vi "Disabled.vi"(7 "Robot Mode":T2, 10 "Match Info":T1={"Autonomous Elapsed Seconds"=0.0, "TeleOp Elapsed Seconds"=0.0, "Disabled Elapsed Seconds"=0.0, "Visited Autonomous"=FALSE, "Visited TeleOp"=FALSE, "Visited Disabled"=FALSE, "Autonomous Settings"={"Autonomous Style"=enum."Independent", "VI Refnum"=refnum}}, 11 "Call Context":T3) -> ()   [LabVIEW 2011]
doc: "This VI is called each time a disabled packet is received from the DS. It is often used to prepare for the next robot mode, to calibrate sensors, etc."
uses:
  <vilib>/Rock Robotics/WPI/DriverStation/WPI_DriverStationDerivedRobotMode.ctl
  <vilib>/Rock Robotics/WPI/DriverStation/WPI_DriverStationRobotMode.ctl
  <vilib>/Rock Robotics/WPI/DriverStation/WPI_DriverStationMatch Info.ctl
  <vilib>/Rock Robotics/WPI/DriverStation/DriverStationLCD/WPI_DriverStationLCDLCDLine.ctl
  <vilib>/Rock Robotics/WPI/CAN/Jaguar/SubVIs/WPI_CANJaguar_ControlMode.ctl
  <vilib>/Rock Robotics/WPI/MotorControl/WPI_MotorControlDeviceRef.ctl
  <vilib>/Rock Robotics/SystemInterfaces/Typedef/FPGA_TypedefDigitalModule.ctl
  <vilib>/Rock Robotics/SystemInterfaces/DIO/FPGA_DIOPWMChannel.ctl
  <vilib>/Rock Robotics/WPI/PWM/WPI_PWMDeadband.ctl
  <vilib>/Rock Robotics/WPI/PWM/WPI_PWMTransform_ConPane.ctl
  <vilib>/Utility/file.llb/Read From Spreadsheet File (string).vi
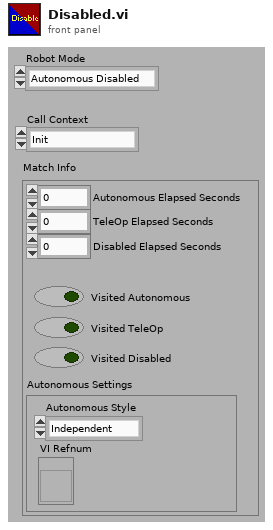
[diagram p1: front panel]
types:
  T1 = typedef "WPI_DriverStationMatch Info.ctl" = cluster{"Autonomous Elapsed Seconds":dbl, "TeleOp Elapsed Seconds":dbl, "Disabled Elapsed Seconds":dbl, "Visited Autonomous":bool, "Visited TeleOp":bool, "Visited Disabled":bool, "Autonomous Settings":cluster{"Autonomous Style":enum16{"Iterative", "Independent"}, "VI Refnum":refnum<vi>}}
  T2 = typedef "WPI_DriverStationRobotMode.ctl" = enum16{"Autonomous Disabled", "Autonomous Enabled", "Teleop Disabled", "Teleop Enabled", "Timeout", "Finish"}
  T3 = typedef "WPI_DriverStationDerivedRobotMode.ctl" = enum16{"Init", "Execute", "Stop"}
  T4 = typedef "WPI_MotorControlDeviceRef.ctl" = cluster{"DeviceStatus":errorcluster, "Type":enum16{"PWM", "CAN"}, "PWM":cluster{"Digital Module":T5, "PWM Channel":T6, "DeadBand":T7}, "CAN":cluster{"Device Number":u8, "Control Mode":T8, "Semaphore":T9, "Max Vout":dbl}, "Invert":bool, "TransformRef":T10, "InvTransformRef":T10}
  T5 = typedef "FPGA_TypedefDigitalModule.ctl" = enum16{"Digital Module 1", "Digital Module 2"}
  T6 = typedef "FPGA_DIOPWMChannel.ctl" = enum8{"PWM 1", "PWM 2", "PWM 3", "PWM 4", "PWM 5", "PWM 6", "PWM 7", "PWM 8", "PWM 9", "PWM 10", "Invalid"}
  T7 = typedef "WPI_PWMDeadband.ctl" = cluster{"Name":string, "maxPositivePwm":i32, "minPositivePwm":i32, "centerPwm":i32, "maxNegativePwm":i32, "minNegativePwm":i32, "angularRange":u16}
  T8 = typedef "WPI_CANJaguar_ControlMode.ctl" = enum8{"Percent VBus", "Current", "Speed", "Position", "Voltage"}
  T9 = typedef "Semaphore RefNum" = refnum<k1>
  T10 = typedef "WPI_PWMTransform_ConPane.ctl" = refnum<vi>
  T11 = typedef "WPI_DriverStationLCDLCDLine.ctl" = enum16{"Main - Line 1", "User - Line 2", "User - Line 3", "User - Line 4", "User - Line 5", "User - Line 6"}
  T12 = typedef "WPI_JoystickDevRef.ctl" = cluster{"Device":T13}
  T13 = typedef "WPI_JoystickDeviceEnum.ctl" = enum16{"USB 1", "USB 2", "USB 3", "USB 4", "Kinect 1", "Kinect 2"}
  T14 = typedef "WPI_JoystickButtonState.ctl" = cluster{"Button 1":bool, "Button 2":bool, "Button 3":bool, "Button 4":bool, "Button 5":bool, "Button 6":bool, "Button 7":bool, "Button 8":bool, "Button 9":bool, "Button 10":bool, "Button 11":bool, "Button 12":bool}
  T15 = cluster{"axis 1 (x)":dbl, "axis 2 (y)":dbl, "axis 3 (throttle)":dbl, "axis 4":dbl, "axis 5":dbl, "axis 6":dbl}
  T16 = typedef "IMAQ Image.ctl" = refnum<image>
  T17 = enum32{"Gray", "Binary", "Gradient", "Rainbow", "Temperature"}
  T18 = typedef "WPI_CameraDevRef.ctl" = cluster{"Camera Address":string, "CameraStatus":errorcluster, "Acquire Image Notifier":refnum<notifier>}
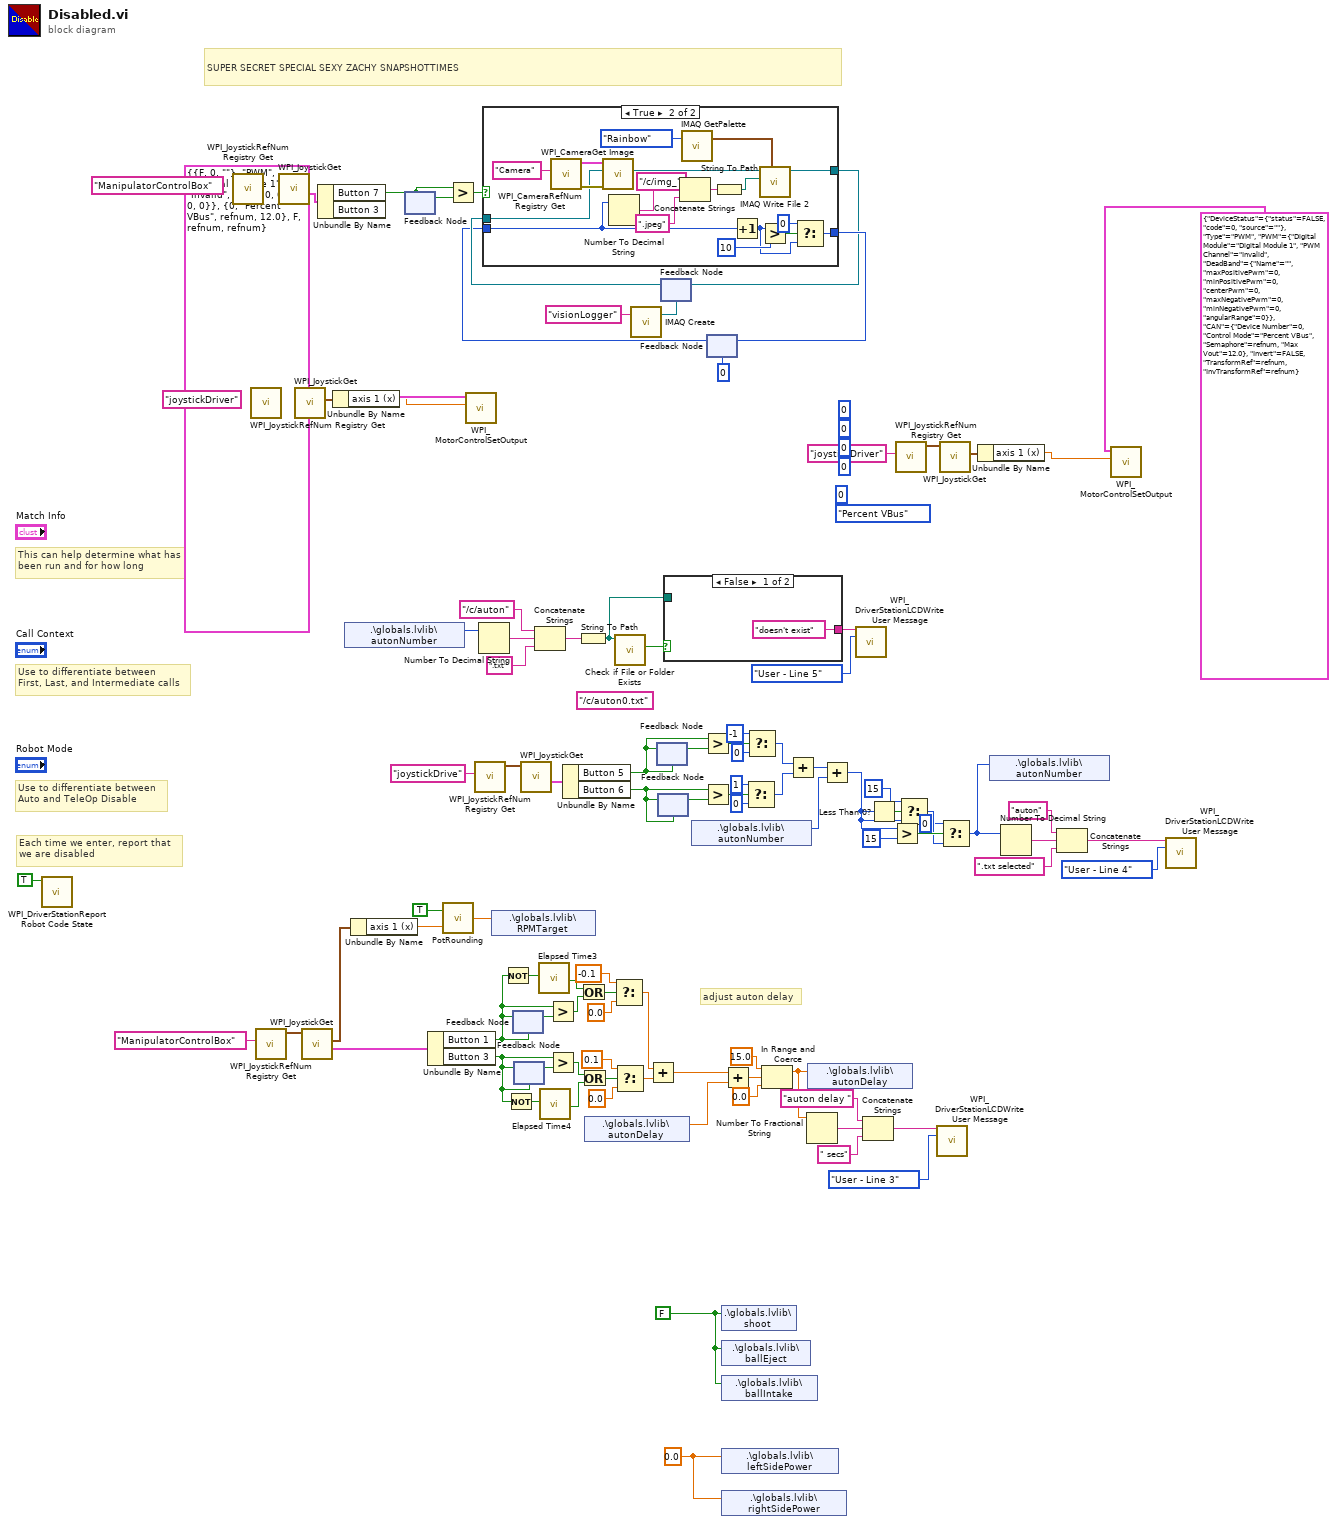
[diagram p0: block diagram]
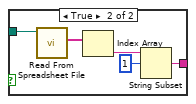
[diagram p3: hidden frame]
diagram:
  (unwired) 0 ("centerPwm")
  (unwired) 0 ("maxNegativePwm")
  (unwired) 0 ("minNegativePwm")
  (unwired) u16 0 ("angularRange")
  (unwired) u8 0 ("Device Number")
  (unwired) WPI_CANJaguar_ControlMode."Percent VBus" ("Control Mode")
  w29 = 0.0 ("leftSidePower")
  (unwired) "/c/auton0.txt" ("f")
  w100 = FALSE ("shoot")
  # "SUPER SECRET SPECIAL SEXY ZACHY SNAPSHOTTIMES"
  # "adjust auton delay"
  # "Each time we enter, report that\nwe are disabled"
  # "Use to differentiate between\nFirst, Last, and Intermediate calls"
  # "This can help determine what has\nbeen run and for how long"
  # "Use to differentiate between\nAuto and TeleOp Disable"
  n1 = call <vilib>:"WPI_DriverStationReport Robot Code State.vi"("Disabled"=TRUE ("Autonomous")) -> ()  [unwired: 10 in, 1 out]
  n2 = call <vilib>:"WPI_JoystickRefNum Registry Get.vi"("refnum name"="ManipulatorControlBox") -> ("JoystickDevRef"=w17:T12)  [unwired: 9 in, 1 out]
  n3 = call <vilib>:"WPI_JoystickRefNum Registry Get.vi"("refnum name"="joystickDriver") -> ("JoystickDevRef"=w9:T12)  [unwired: 9 in, 1 out]
  n4 = call <vilib>:"WPI_JoystickRefNum Registry Get.vi"("refnum name"="ManipulatorControlBox") -> ("JoystickDevRef"=w66:T12)  [unwired: 9 in, 1 out]
  n5 = call <vilib>:"WPI_JoystickGet.vi"("JoystickDevRef"=w17) -> ("Buttons"=w15:T14)  [unwired: 4 in, 2 out]
  n6 = call <vilib>:"WPI_JoystickGet.vi"("JoystickDevRef"=w9) -> ("Axes"=w8:T15)  [unwired: 4 in, 2 out]
  n7 = call <vilib>:"WPI_JoystickGet.vi"("JoystickDevRef"=w66) -> ("Buttons"=w68:T14, "Axes"=w30:T15)  [unwired: 4 in, 1 out]
  n8 = Unbundle By Name(w15) -> ("Button 7"=w13:bool)  [unwired: 1 out]
  n9 = Unbundle By Name(w8) -> ("axis 1 (x)"=w6:dbl)
  n10 = shared-variable ".\\globals.lvlib\\autonNumber"() -> (w99:i8)  [unwired: 1 in, 1 out]
  n11 = Unbundle By Name(w30) -> ("axis 1 (x)"=w32:dbl)
  n12 = feedback #1() -> (w14:bool)  [unwired: 1 in]
  n13 = feedback-in #1(w13) -> ()
  n14 = Unbundle By Name(w68) -> ("Button 1"=w64:bool, "Button 3"=w72:bool)
  n15 = call "PotRounding.vi"("Potentiometer"=w32, "Invert?"=TRUE) -> ("shooter output"=w28:dbl)
  n16 = Greater?(x=w13, y=w14) -> (0:w12:bool)
  n17 = call <vilib>:"WPI_MotorControlSetOutput.vi"("Output"=w6, "MotorControlDevRef"=T4 {"DeviceStatus"={"status"=FALSE, "code"=0, "source"=""}, "Type"=enum."PWM", "PWM"={"Digital Module"=enum."Digital Module 1", "PWM Channel"=enum."Invalid", "DeadBand"={"Name"="", "maxPositivePwm"=0, "minPositivePwm"=0, "centerPwm"=0, "maxNegativePwm"=0, "minNegativePwm"=0, "angularRange"=0}}, "CAN"={"Device Number"=0, "Control Mode"=enum."Percent VBus", "Semaphore"=refnum, "Max Vout"=12.0}, "Invert"=FALSE, "TransformRef"=refnum, "InvTransformRef"=refnum}) -> ()  [unwired: 8 in, 2 out]
  n18 = call <vilib>:"WPI_JoystickRefNum Registry Get.vi"("refnum name"="joystickDrive") -> ("JoystickDevRef"=w62:T12)  [unwired: 9 in, 1 out]
  n19 = Number To Decimal String(number=w99) -> (decimal integer string=w97:string)  [unwired: 1 in]
  n20 = shared-variable ".\\globals.lvlib\\RPMTarget"(w28) -> ()  [unwired: 1 in, 1 out]
  n21 = Not(x=w64) -> (.not. x?=w65:bool)
  n22 = Not(x=w72) -> (.not. x?=w71:bool)
  n23 = feedback #2(w64) -> (w69:bool)
  n24 = feedback-in #2(w64) -> ()
  n25 = feedback #3(w72) -> (w70:bool)
  n26 = feedback-in #3(w72) -> ()
  n27 = call <vilib>:"WPI_JoystickGet.vi"("JoystickDevRef"=w62) -> ("Buttons"=w60:T14)  [unwired: 4 in, 2 out]
  n28 = Concatenate Strings("/c/auton", w97, ".txt" ("string")) -> (w95:string)
  n29 = call "Elapsed Time3"("Reset"=w65) -> ("Time has Elapsed"=w80:bool)  [unwired: 11 in, 7 out]
  n30 = call "Elapsed Time4"("Reset"=w71) -> ("Time has Elapsed"=w74:bool)  [unwired: 11 in, 7 out]
  n31 = Greater?(x=w64, y=w69) -> (0:w81:bool)
  n32 = Greater?(x=w72, y=w70) -> (0:w73:bool)
  n33 = Unbundle By Name(w60) -> ("Button 5"=w52:bool, "Button 6"=w51:bool)
  n34 = String To Path(string=w95) -> (path=w24:path)
  n35 = Or(x=w80, y=w81) -> (x .or. y?=w79:bool)
  n36 = Or(x=w73, y=w74) -> (x .or. y?=w75:bool)
  n37 = shared-variable ".\\globals.lvlib\\autonDelay"() -> (w85:dbl)  [unwired: 1 in, 1 out]
  n38 = Select(t=-0.1, s=w79, f=0.0 ("t")) -> (s? t:f=w82:dbl)
  n39 = call <vilib>:"Check if File or Folder Exists.vi"("path"=w24) -> ("file or folder exists?"=w27:bool)  [unwired: 8 in, 2 out]
  n40 = Select(t=0.1, s=w75, f=0.0 ("t")) -> (s? t:f=w83:dbl)
  n41 = call "IMAQ Create"("Image Name"="visionLogger") -> ("New Image"=w23:T16)  [unwired: 4 in, 1 out]
  n42 = Add(x=w82, y=w83) -> (x+y=w84:dbl)
  n43 = feedback #4(w52) -> (w58:bool)
  n44 = feedback-in #4(w52) -> ()
  n45 = feedback #5(w51) -> (w57:bool)
  n46 = feedback-in #5(w51) -> ()
  n47 = feedback #6(w23) -> (w21:T16)
  n48 = case shown="False" w27 {
    tunnel: ["doesn't exist" ("String") w104] -> w25
    tunnel: w24 -> [_ w103]
    frame False {
    }
    frame True {
      n49 = call-poly <vilib>:"Read From Spreadsheet File.vi"("file path (dialog if empty)"=w103) -> ("first row"=w107:string[])  [unwired: 6 in, 4 out]
      n50 = Index Array(array=w107) -> (element=w106:string)  [unwired: 1 in]
      n51 = String Subset(string=w106, offset (0)=1) -> (substring=w104:string)  [unwired: 1 in]
    }
  }
  n52 = shared-variable ".\\globals.lvlib\\autonNumber"() -> (w42:i8)  [unwired: 1 in, 1 out]
  n53 = Greater?(x=w52, y=w58) -> (0:w44:bool)
  n54 = Greater?(x=w51, y=w57) -> (0:w45:bool)
  n55 = feedback #7(0) -> (w19:i32)
  n56 = case shown="True" w12 {
    tunnel: w21 -> [w108 w122]
    tunnel: [w109 w115] -> w20
    tunnel: w19 -> [w109 w112]
    tunnel: [w108 w121] -> w18
    frame False {
    }
    frame True {
      n57 = call <vilib>:"WPI_CameraRefNum Registry Get.vi"("refnum name"="Camera") -> ("error out"=w127:errorcluster, "CameraDevRef"=w126:T18)  [unwired: 9 in]
      n58 = call <vilib>:"WPI_CameraGet Image.vi"("error in (no error)"=w127, "Image"=w122, "CameraDevRef"=w126) -> ("Image Out"=w125:T16)  [unwired: 6 in, 2 out]
      n59 = Number To Decimal String(number=w112) -> (decimal integer string=w119:string)  [unwired: 1 in]
      n60 = Concatenate Strings("/c/img_", w119, ".jpeg" ("string")) -> (w116:string)
      n61 = call "IMAQ GetPalette"("Palette Number (gray)"=T17."Rainbow") -> ("Color Palette"=w124:cluster{"Red":u8, "Green":u8, "Blue":u8}[])  [unwired: 4 in, 1 out]
      n62 = String To Path(string=w116) -> (path=w117:path)
      n63 = Increment(x=w112) -> (x+1=w110:i32)
      n64 = call-poly "IMAQ Write File 2"("Color Palette"=w124, "File Path"=w117, "Image"=w125) -> ("Image Out (duplicate)"=w121:T16)  [unwired: 7 in, 1 out]
      n65 = Greater?(x=w110, y=10) -> (0:w114:bool)
      n66 = Select(t=0, s=w114, f=w110) -> (s? t:f=w115:i32)
    }
  }
  n67 = feedback-in #6(w18) -> ()
  n68 = feedback-in #7(w20) -> ()
  n69 = shared-variable ".\\globals.lvlib\\shoot"(w100) -> ()  [unwired: 1 in, 1 out]
  n70 = shared-variable ".\\globals.lvlib\\ballEject"(w100) -> ()  [unwired: 1 in, 1 out]
  n71 = shared-variable ".\\globals.lvlib\\ballIntake"(w100) -> ()  [unwired: 1 in, 1 out]
  n72 = shared-variable ".\\globals.lvlib\\leftSidePower"(w29) -> ()  [unwired: 1 in, 1 out]
  n73 = shared-variable ".\\globals.lvlib\\rightSidePower"(w29) -> ()  [unwired: 1 in, 1 out]
  n74 = Add(x=w84, y=w85) -> (x+y=w86:dbl)
  n75 = Select(t=i8 1, s=w45, f=i8 0 ("t")) -> (s? t:f=w53:i8)
  n76 = Select(t=i8 -1, s=w44, f=i8 0 ("t")) -> (s? t:f=w54:i8)
  n77 = In Range and Coerce(upper limit=15.0, x=w86, lower limit=0.0) -> (coerced(x)=w89:dbl)  [unwired: 1 out]
  n78 = Add(x=w54, y=w53) -> (x+y=w43:i8)
  n79 = Number To Fractional String(number=w89) -> (F-format string=w90:string)  [unwired: 3 in]
  n80 = shared-variable ".\\globals.lvlib\\autonDelay"(w89) -> ()  [unwired: 1 in, 1 out]
  n81 = Add(x=w43, y=w42) -> (x+y=w38:i8)
  n82 = call <vilib>:"WPI_DriverStationLCDWrite User Message.vi"("line text"=w25, "line"=WPI_DriverStationLCDLCDLine."User - Line 5") -> ()  [unwired: 13 in, 1 out]
  n83 = Concatenate Strings("auton delay " ("string"), w90, " secs" ("string")) -> (w93:string)
  n84 = Less Than 0?(x=w38) -> (x < 0?=w40:bool)
  n85 = Greater?(x=w38, y=i8 15) -> (0:w36:bool)
  n86 = call <vilib>:"WPI_JoystickRefNum Registry Get.vi"("refnum name"="joystickDriver") -> ("JoystickDevRef"=w4:T12)  [unwired: 9 in, 1 out]
  n87 = Select(t=i8 15, s=w40, f=w38) -> (s? t:f=w35:i8)
  n88 = call <vilib>:"WPI_DriverStationLCDWrite User Message.vi"("line text"=w93, "line"=WPI_DriverStationLCDLCDLine."User - Line 3") -> ()  [unwired: 13 in, 1 out]
  n89 = call <vilib>:"WPI_JoystickGet.vi"("JoystickDevRef"=w4) -> ("Axes"=w3:T15)  [unwired: 4 in, 2 out]
  n90 = Select(t=i8 0, s=w36, f=w35) -> (s? t:f=w33:i8)
  n91 = Unbundle By Name(w3) -> ("axis 1 (x)"=w2:dbl)
  n92 = shared-variable ".\\globals.lvlib\\autonNumber"(w33) -> ()  [unwired: 1 in, 1 out]
  n93 = Number To Decimal String(number=w33) -> (decimal integer string=w50:string)  [unwired: 1 in]
  n94 = Concatenate Strings("auton" ("string"), w50, ".txt selected" ("string")) -> (w47:string)
  n95 = call <vilib>:"WPI_MotorControlSetOutput.vi"("Output"=w2, "MotorControlDevRef"=T4 {"DeviceStatus"={"status"=FALSE, "code"=0, "source"=""}, "Type"=enum."PWM", "PWM"={"Digital Module"=enum."Digital Module 1", "PWM Channel"=enum."Invalid", "DeadBand"={"Name"="", "maxPositivePwm"=0, "minPositivePwm"=0, "centerPwm"=0, "maxNegativePwm"=0, "minNegativePwm"=0, "angularRange"=0}}, "CAN"={"Device Number"=0, "Control Mode"=enum."Percent VBus", "Semaphore"=refnum, "Max Vout"=12.0}, "Invert"=FALSE, "TransformRef"=refnum, "InvTransformRef"=refnum}) -> ()  [unwired: 8 in, 2 out]
  n96 = call <vilib>:"WPI_DriverStationLCDWrite User Message.vi"("line text"=w47, "line"=WPI_DriverStationLCDLCDLine."User - Line 4") -> ()  [unwired: 13 in, 1 out]
